vi "Interface_Dispatch_Initialize Module.vi"(8 "error in (no error)":errorcluster, 11 "Dispatch_Demand Limiting in":refnum<class "Dispatch_Demand Limiting.lvclass">) -> (0 "error out":errorcluster, 2 "TagDescriptions":refnum<class "tag descriptor.lvclass">[](array[class]), 3 "Dispatch_Demand Limiting out":refnum<class "Dispatch_Demand Limiting.lvclass">)   [LabVIEW 2015, in "Dispatch_Demand Limiting.lvclass"]
uses:
  Dispatch_Demand Limiting.lvclass
  <vilib>/NI/Tag Bus/tag/tag descriptor.lvclass
  TagBus/TagBus.lvclass
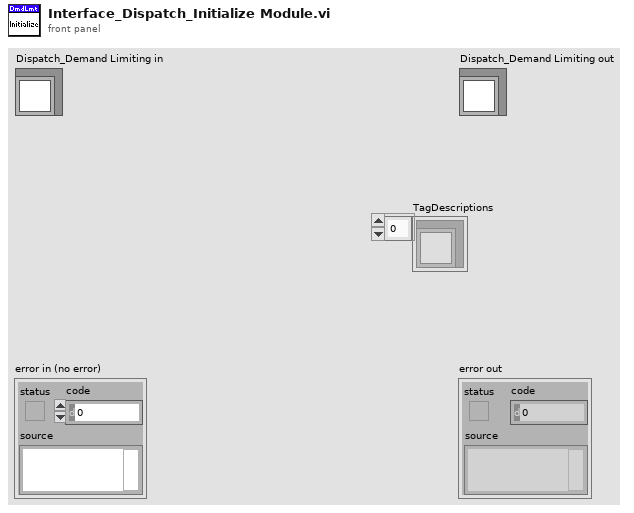
[diagram p1: front panel]
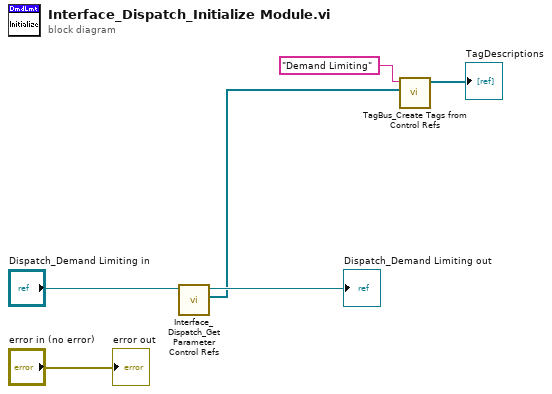
[diagram p0: block diagram]
diagram:
  n1 = call-dynamic "Interface_Dispatch_Get Parameter Control Refs.vi"("Dispatch_Demand Limiting in"="Dispatch_Demand Limiting in") -> ("Configuration Controls[]"=w3:refnum<vi>[], "Dispatch_Demand Limiting out"=→"Dispatch_Demand Limiting out":refnum<class "Dispatch_Demand Limiting.lvclass">)  [unwired: 6 in, 3 out]
  n2 = call "TagBus_Create Tags from Control Refs.vi"("Array"=w3, "Prepend Tag Name"="Demand Limiting" ("Process Name")) -> ("TagDescriptions"=→"TagDescriptions":refnum<class "tag descriptor.lvclass">[])  [unwired: 9 in]
  "error out" <- "error in (no error)"
